vi "PowerSupply.vi"   [LabVIEW 2016]
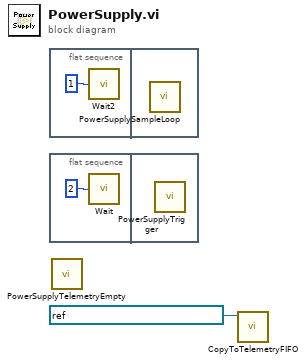
[diagram p0: block diagram]
diagram:
  n1 = flat-sequence {
    frame #0 {
      n2 = call "Wait2"("Count(mSec)"=u8 1) -> ()  [unwired: 1 out]
    }
    frame #1 {
      n3 = call "PowerSupplySampleLoop.vi"() -> ()  [unwired: 12 in]
    }
  }
  n4 = flat-sequence {
    frame #0 {
      n5 = call "Wait"("Count(mSec)"=u8 2) -> ()  [unwired: 1 out]
    }
    frame #1 {
      n6 = call "PowerSupplyTrigger.vi"() -> ()  [unwired: 12 in]
    }
  }
  n7 = call "PowerSupplyTelemetryEmpty.vi"() -> ()  [unwired: 12 in]
  n8 = call "CopyToTelemetryFIFO.vi"("SourceFIFO"=refnum<k21> "PowerSupplyTelemetryFIFO") -> ()  [unwired: 11 in]
